vi "Histogram Grid Comparison.vi"(8 "error in":errorcluster, 10 "Image 2":path, 11 "Image 1":path) -> (0 "error out":errorcluster, 2 "Histogram Graphs":T1(array[cluster]), 3 "Histogram Grid Comparison Score":dbl)   [LabVIEW 2014, in "Histogram Grid Comparison.lvclass"]
uses:
  Histogram Grid Comparison.lvclass
  Image Comparison/Image Comparison.lvclass
  <vilib>/Analysis/NI_AALBase.lvlib
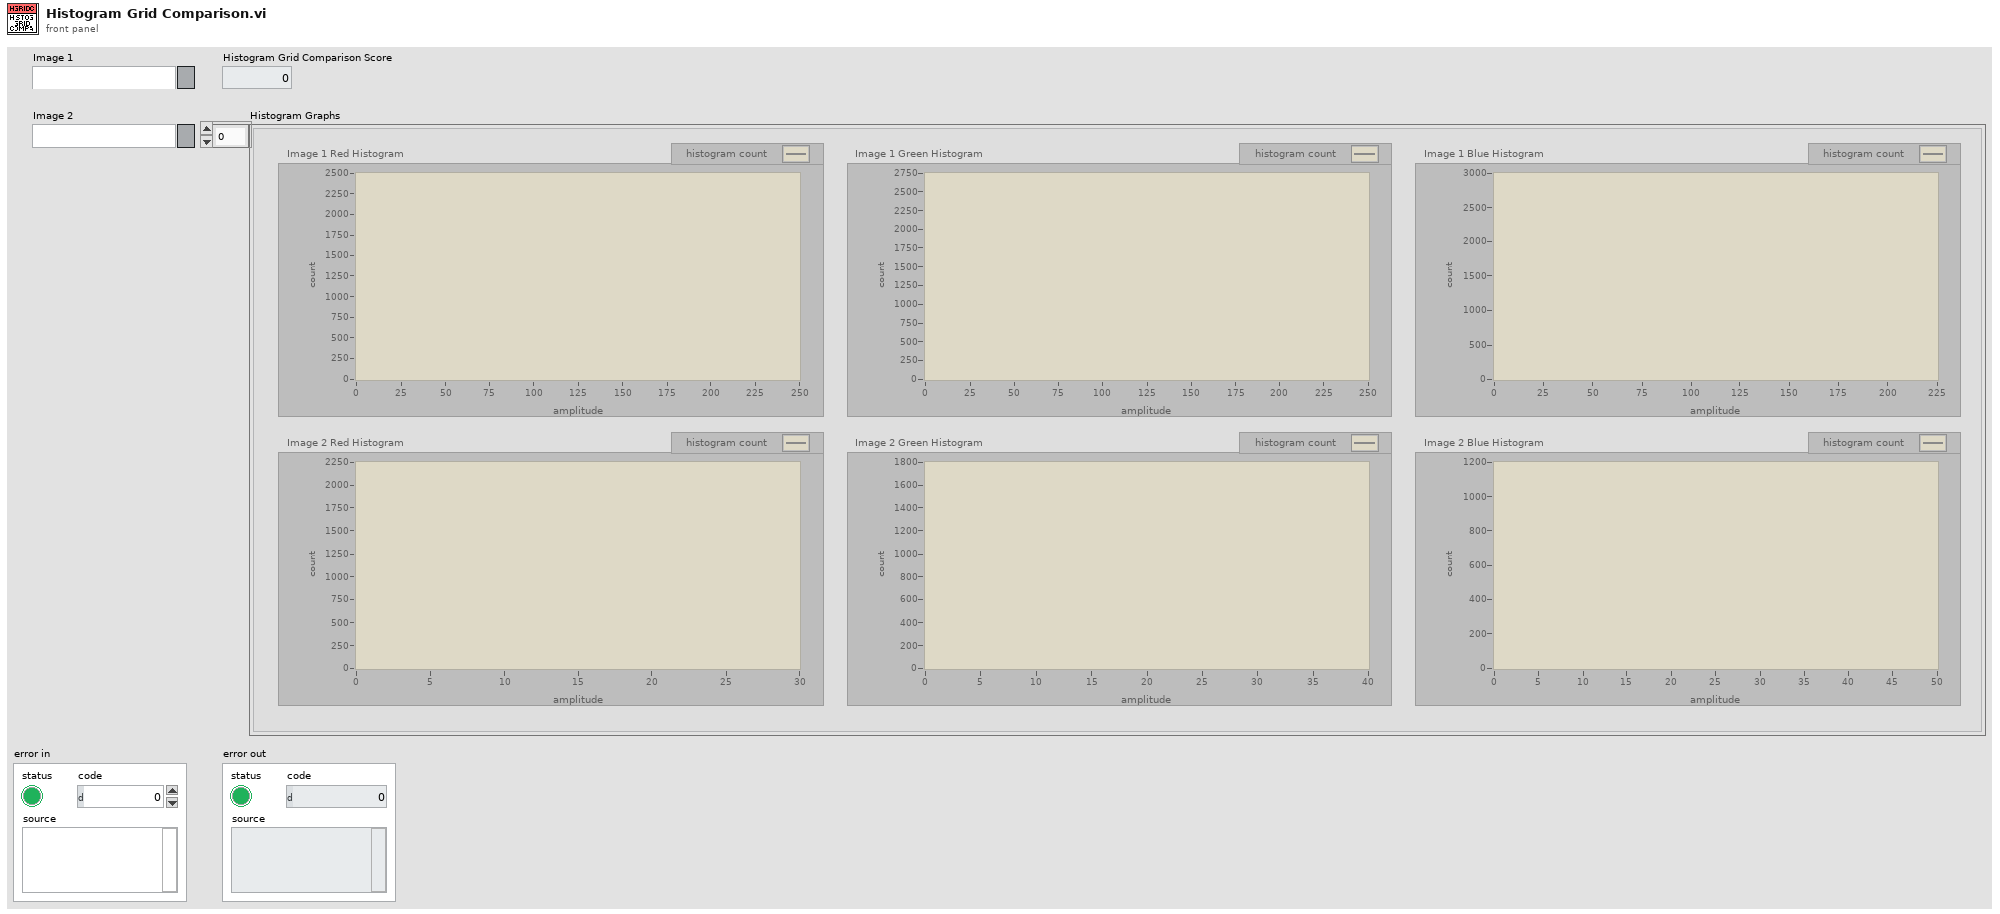
[diagram p1: front panel]
types:
  T1 = cluster{"Image 1 Red Histogram":cluster{"X Values":dbl[], "Histogram: h(x)":i32[]}, "Image 1 Green Histogram":cluster{"X Values":dbl[], "Histogram: h(x)":i32[]}, "Image 1 Blue Histogram":cluster{"X Values":dbl[], "Histogram: h(x)":i32[]}, "Image 2 Red Histogram":cluster{"X Values":dbl[], "Histogram: h(x)":i32[]}, "Image 2 Green Histogram":cluster{"X Values":dbl[], "Histogram: h(x)":i32[]}, "Image 2 Blue Histogram":cluster{"X Values":dbl[], "Histogram: h(x)":i32[]}}[]
  T2 = typedef "imagedata.ctl" = cluster{"image type":i32, "image depth":i32, "image":u8[], "mask":u8[], "colors":u32[], "Rectangle":cluster{"left":i16, "top":i16, "right":i16, "bottom":i16}}
  T3 = cluster{"Image 1 Red Histogram":cluster{"X Values":dbl[], "Histogram: h(x)":i32[]}, "Image 1 Green Histogram":cluster{"X Values":dbl[], "Histogram: h(x)":i32[]}, "Image 1 Blue Histogram":cluster{"X Values":dbl[], "Histogram: h(x)":i32[]}, "Image 2 Red Histogram":cluster{"X Values":dbl[], "Histogram: h(x)":i32[]}, "Image 2 Green Histogram":cluster{"X Values":dbl[], "Histogram: h(x)":i32[]}, "Image 2 Blue Histogram":cluster{"X Values":dbl[], "Histogram: h(x)":i32[]}}
  T4 = cluster{"X Values":dbl[], "Histogram: h(x)":i32[]}
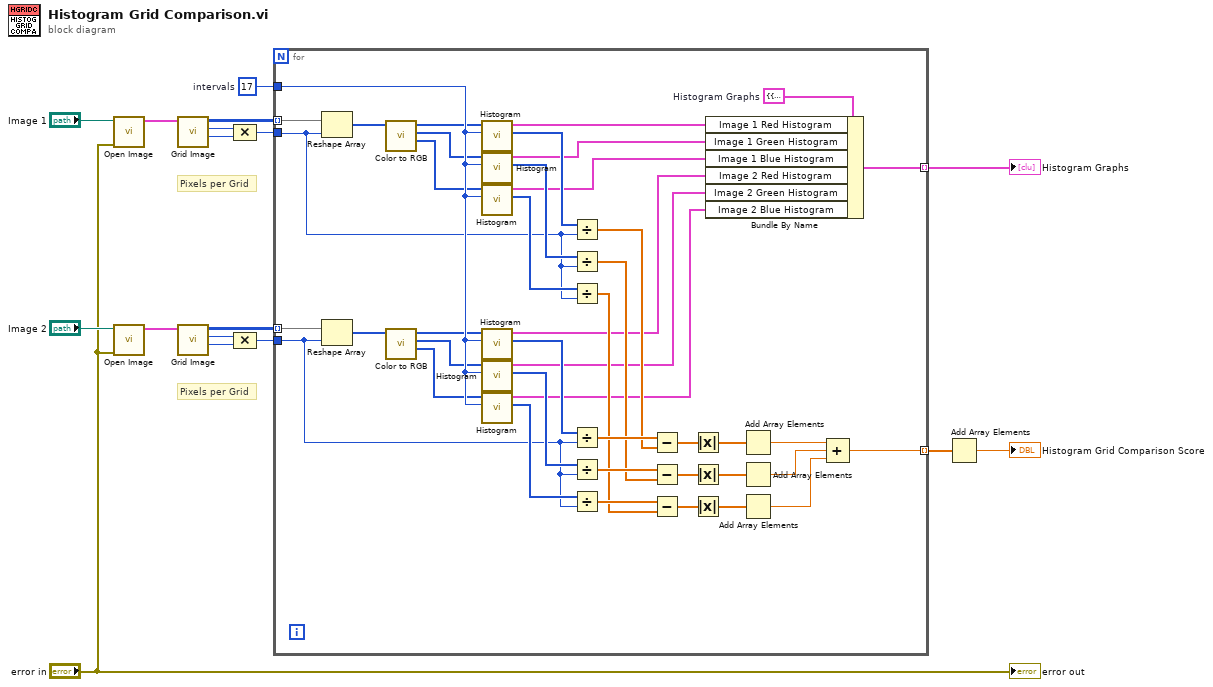
[diagram p0: block diagram]
diagram:
  w4 = 17  # intervals
  # "Pixels per Grid"
  # "Pixels per Grid"
  n1 = call "Open Image.vi"("error in (no error)"="error in", "Image"="Image 1") -> ("image data"=w16:T2)  [unwired: 8 in, 1 out]
  n2 = call "Open Image.vi"("error in (no error)"="error in", "Image"="Image 2") -> ("image data"=w14:T2)  [unwired: 8 in, 1 out]
  n3 = call "Grid Image.vi"("image data"=w16) -> ("Vertical Grid Size"=w10:i32, "Horizontal Grid Size"=w11:i32, "Grid of 2D Pixel Arrays"=w12:u32[][][])  [unwired: 6 in, 2 out]
  n4 = call "Grid Image.vi"("image data"=w14) -> ("Vertical Grid Size"=w7:i32, "Horizontal Grid Size"=w8:i32, "Grid of 2D Pixel Arrays"=w13:u32[][][])  [unwired: 6 in, 2 out]
  n5 = Compound Arithmetic op=MULTIPLY(w11, w10) -> (w9:i32)
  n6 = Compound Arithmetic op=MULTIPLY(w8, w7) -> (w6:i32)
  n7 = for {
    tunnel: w13 -> [w58] mode=indexing
    tunnel: w12 -> [w59] mode=indexing
    tunnel: w9 -> [w43]
    tunnel: w6 -> [w42]
    tunnel: w4 -> [w60]
    tunnel: [w26] -> w3 mode=indexing
    tunnel: [w18] -> w1 mode=indexing
    w25 = T3 {"Image 1 Red Histogram"={"X Values"=[], "Histogram: h(x)"=[]}, "Image 1 Green Histogram"={"X Values"=[], "Histogram: h(x)"=[]}, "Image 1 Blue Histogram"={"X Values"=[], "Histogram: h(x)"=[]}, "Image 2 Red Histogram"={"X Values"=[], "Histogram: h(x)"=[]}, "Image 2 Green Histogram"={"X Values"=[], "Histogram: h(x)"=[]}, "Image 2 Blue Histogram"={"X Values"=[], "Histogram: h(x)"=[]}}  # Histogram Graphs
    n8 = Reshape Array(w59, w43) -> (w57:u32[])
    n9 = Reshape Array(w58, w42) -> (w56:u32[])
    n10 = call "Color to RGB.vi"("1D Pixel Array"=w57) -> ("Blue[]"=w53:u8[], "Green[]"=w54:u8[], "Red[]"=w55:u8[])  [unwired: 8 in]
    n11 = call "Color to RGB.vi"("1D Pixel Array"=w56) -> ("Blue[]"=w50:u8[], "Green[]"=w51:u8[], "Red[]"=w52:u8[])  [unwired: 8 in]
    n12 = call <vilib>:"Histogram.vi"("intervals"=w60, "X"=w55) -> ("Histogram: h(x)"=w49:i32[], "Histogram Graph"=w24:T4)  [unwired: 6 in, 2 out]
    n13 = call <vilib>:"Histogram.vi"("intervals"=w60, "X"=w54) -> ("Histogram: h(x)"=w48:i32[], "Histogram Graph"=w23:T4)  [unwired: 6 in, 2 out]
    n14 = call <vilib>:"Histogram.vi"("intervals"=w60, "X"=w53) -> ("Histogram: h(x)"=w47:i32[], "Histogram Graph"=w22:T4)  [unwired: 6 in, 2 out]
    n15 = call <vilib>:"Histogram.vi"("intervals"=w60, "X"=w52) -> ("Histogram: h(x)"=w46:i32[], "Histogram Graph"=w21:T4)  [unwired: 6 in, 2 out]
    n16 = call <vilib>:"Histogram.vi"("intervals"=w60, "X"=w51) -> ("Histogram: h(x)"=w45:i32[], "Histogram Graph"=w20:T4)  [unwired: 6 in, 2 out]
    n17 = call <vilib>:"Histogram.vi"("intervals"=w60, "X"=w50) -> ("Histogram: h(x)"=w44:i32[], "Histogram Graph"=w19:T4)  [unwired: 6 in, 2 out]
    n18 = Divide(x=w49, y=w43) -> (x/y=w40:dbl[])
    n19 = Divide(x=w48, y=w43) -> (x/y=w38:dbl[])
    n20 = Divide(x=w47, y=w43) -> (x/y=w36:dbl[])
    n21 = Divide(x=w46, y=w42) -> (x/y=w41:dbl[])
    n22 = Divide(x=w45, y=w42) -> (x/y=w39:dbl[])
    n23 = Divide(x=w44, y=w42) -> (x/y=w37:dbl[])
    n24 = Subtract(x=w41, y=w40) -> (x-y=w29:dbl[])
    n25 = Subtract(x=w39, y=w38) -> (x-y=w28:dbl[])
    n26 = Subtract(x=w37, y=w36) -> (x-y=w27:dbl[])
    n27 = Absolute Value(x=w29) -> (abs(x)=w35:dbl[])
    n28 = Absolute Value(x=w28) -> (abs(x)=w34:dbl[])
    n29 = Absolute Value(x=w27) -> (abs(x)=w33:dbl[])
    n30 = Bundle By Name(cluster=w25, "Image 1 Red Histogram"=w24, "Image 1 Green Histogram"=w23, "Image 1 Blue Histogram"=w22, "Image 2 Red Histogram"=w21, "Image 2 Green Histogram"=w20, "Image 2 Blue Histogram"=w19) -> (w18:T3)
    n31 = Add Array Elements(numeric array=w35) -> (sum=w32:dbl)
    n32 = Add Array Elements(numeric array=w34) -> (sum=w31:dbl)
    n33 = Add Array Elements(numeric array=w33) -> (sum=w30:dbl)
    n34 = Compound Arithmetic op=ADD(w32, w31, w30) -> (w26:dbl)
  }
  "Histogram Graphs" <- w1
  n35 = Add Array Elements(numeric array=w3) -> (sum=→"Histogram Grid Comparison Score":dbl)
  "error out" <- "error in"
